vi "WPI_CameraGet White Balance.vi"(8 "error in (no error)":errorcluster, 11 "CameraDevRef":T1={"Camera Address"="192.168.0.90", "CameraStatus"={"status"=FALSE, "code"=0, "source"=""}}) -> (0 "error out":errorcluster, 1 "Color Temp (K)":dbl, 2 "White Balance":T2, 3 "CameraDevRef Out":T1)   [LabVIEW 2017]
doc: "Returns the white balance setting of the camera you specify.\n\nThis software is licensed. Open the labview\\readme\\WPI Robotics Library Open Source License.txt file for more information."
uses:
  <vilib>/Rock Robotics/WPI/Camera/WPI_CameraWhite Balance Values.ctl
  <vilib>/Rock Robotics/WPI/Camera/WPI_CameraDevRef.ctl
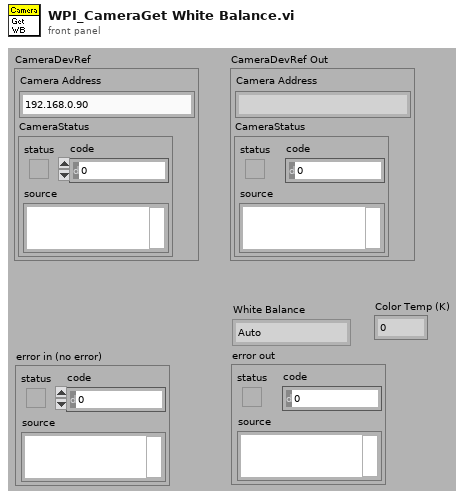
[diagram p1: front panel]
types:
  T1 = typedef "WPI_CameraDevRef.ctl" = cluster{"Camera Address":string, "CameraStatus":errorcluster}
  T2 = typedef "WPI_CameraWhite Balance Values.ctl" = enum16{"Auto", "Fixed indoor", "Fixed outdoor 1", "Fixed outdoor 2", "Fixed fluorescent 1", "Fixed fluorescent 2", "Hold current", "Custom"}
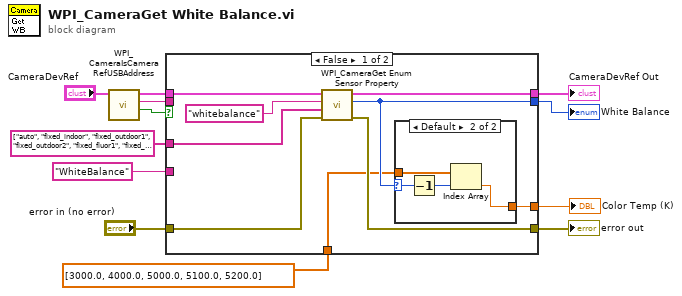
[diagram p0: block diagram]
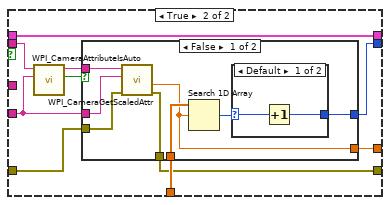
[diagram p3: hidden frame]
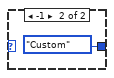
[diagram p4: hidden frame]
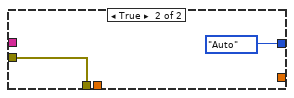
[diagram p5: hidden frame]
diagram:
  n1 = call <vilib>:"WPI_CameraIsCameraRefUSBAddress.vi"("CameraDevRef"="CameraDevRef") -> ("USB?"=w5:bool, "Camera Address Out"=w6:string, "CameraDevRef out"=w3:T1)  [unwired: 7 in, 1 out]
  n2 = case shown="False" w5 {
    tunnel: "error in (no error)" -> [w21 w27]
    tunnel: [w17 w34] -> w11
    tunnel: [w20 w35] -> w10
    tunnel: [w19 w26] -> w9
    tunnel: w3 -> [w18 w35]
    tunnel: w6 -> [_ w33]
    tunnel: "WhiteBalance" -> [_ w28]
    tunnel: dbl[] [3000.0, 4000.0, 5000.0, 5100.0, 5200.0] -> [w15 w32]
    tunnel: [w16 w31] -> w7
    tunnel: string[] ["auto", "fixed_indoor", "fixed_outdoor1", "fixed_outdoor2", "fixed_fluor1", "fixed_fluor2", "hold", "fixed_fluor", "fixed_outdoor"] ("Array") -> [w13 _]
    frame False {
      n3 = call <vilib>:"WPI_CameraGet Enum Sensor Property.vi"("error in (no error)"=w21, "Strings"=w13, "Property Name"="whitebalance" ("format string"), "CameraDevRef"=w18) -> ("error out"=w19:errorcluster, "Enum Int Value"=w17:i32, "CameraDevRef out"=w20:T1)  [unwired: 2 in, 3 out]
      n4 = case shown="Default" w17 {
        selector: w17 -> [_ w25]
        tunnel: [_ w23] -> w16
        tunnel: w15 -> [_ w24]
        frame 0 {
        }
        frame Default {
          n5 = Decrement(x=w25) -> (x-1=w22:i32)
          n6 = Index Array(array=w24, index=w22) -> (element=w23:dbl)
        }
      }
    }
    frame True {
      n7 = call <vilib>:"WPI_CameraAttributeIsAuto.vi"("Attr String"=w28, "Camera Address In"=w33) -> ("Auto?"=w30:bool, "Camera Address Out"=w29:string)  [unwired: 8 in]
      n8 = case shown="False" w30 {
        tunnel: [w41 WPI_CameraWhite_Balance_Values."Auto" ("White Balance")] -> w34
        tunnel: w29 -> [w39 _]
        tunnel: w28 -> [w40 _]
        tunnel: w32 -> [w43 _]
        tunnel: [w36 _] -> w31
        tunnel: w27 -> [w38 w47]
        tunnel: [w37 w47] -> w26
        frame False {
          n9 = call <vilib>:"WPI_CameraGetScaledAttr.vi"("error in (no error)"=w38, "Attr String"=w40, "Camera Address In"=w39) -> ("error out"=w37:errorcluster, "Raw"=w36:dbl)  [unwired: 5 in, 2 out]
          n10 = Search 1D Array(1D array=w43, element=w36) -> (index of element=w42:i32)  [unwired: 1 in]
          n11 = case shown="Default" w42 {
            selector: w42 -> [w45 _]
            tunnel: [w44 WPI_CameraWhite_Balance_Values."Custom" ("White Balance")] -> w41
            frame Default {
              n12 = Increment(x=w45) -> (x+1=w44:i32)
            }
            frame -1 {
            }
          }
        }
        frame True {
        }
      }
    }
  }
  "White Balance" <- w11
  "CameraDevRef Out" <- w10
  "error out" <- w9
  "Color Temp (K)" <- w7
